vi "Lookup Command Info.vi"(8 "error in (no error)":errorcluster, 10 "Channel Lookup Info in":T4 {"Refs" format="%.0x"}, 11 "Item Ref in":T1 format="%.0x") -> (0 "error out":errorcluster, 1 "Command Parameters":T2, 2 "Channel Lookup Info out":T4 {"Refs" format="%.0x"}, 3 "Section Ref out":T1 format="%.0x")   [LabVIEW 2015, in "Instrument Addon System Explorer.lvlib"]
uses:
  Instrument Addon System Explorer.lvlib
  Types/Channel Lookup Cluster.ctl
  <vilib>/NI Veristand/Custom Device API/Custom Device Item Ref.ctl
  Shared/Types/Command Parameters.ctl
  Shared/Types/Linked Channel Cluster.ctl
  Shared/Types/FG Control.ctl
  Shared/MetaData Parameters FG.vi
  <vilib>/NI Veristand/Custom Device API/NI VeriStand - Get Item Property.vi
  <vilib>/NI Veristand/Custom Device API/Get Item Property (String).vi
  <vilib>/NI Veristand/Custom Device API/NI VeriStand - Set Item Property.vi
  <vilib>/NI Veristand/Custom Device API/Set Item Property (U32).vi
  <vilib>/NI Veristand/Custom Device API/Set Item Property (String).vi
  <vilib>/NI Veristand/Custom Device API/Set Item Property (String Array).vi
  <vilib>/NI Veristand/Custom Device API/Get Item Property (U32).vi
  <vilib>/NI Veristand/Custom Device API/Get Item Property (String Array).vi
  Shared/Constants.vi
  <vilib>/NI Veristand/Custom Device API/Set Item Property (Boolean).vi
  <vilib>/NI Veristand/Custom Device API/Get Item Property (Boolean).vi
  <vilib>/NI Veristand/Custom Device Tools/Custom Device Utility Library/NI VeriStand - Search for Item by GUID.vi
  <vilib>/NI Veristand/Custom Device Tools/Custom Device Utility Library/Custom Device Utility Library.lvlib
  Shared/Instrument Addon Shared.lvlib
  <vilib>/NI Veristand/Custom Device API/Custom Device API.lvlib
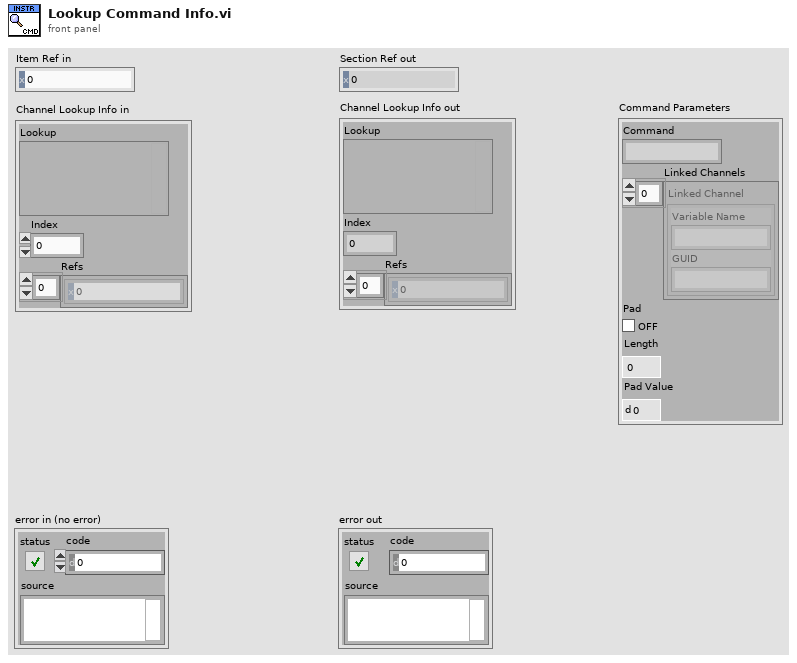
[diagram p1: front panel]
types:
  T1 = typedef "Custom Device API.lvlib/Custom Device Item Ref.ctl" = u64
  T2 = typedef "Instrument Addon Shared.lvlib/Command Parameters.ctl" = cluster{"Command":string, "Linked Channels":T3[], "Pad":bool, "Length":u32, "Pad Value":u8}
  T3 = typedef "Instrument Addon Shared.lvlib/Linked Channel Cluster.ctl" = cluster{"Variable Name":string, "GUID":string}
  T4 = typedef "Instrument Addon System Explorer.lvlib/Channel Lookup Cluster.ctl" = cluster{"Lookup":variant, "Index":i32, "Refs":T1[]}
  T5 = typedef "Instrument Addon Shared.lvlib/FG Control.ctl" = enum16{"Get", "Set"}
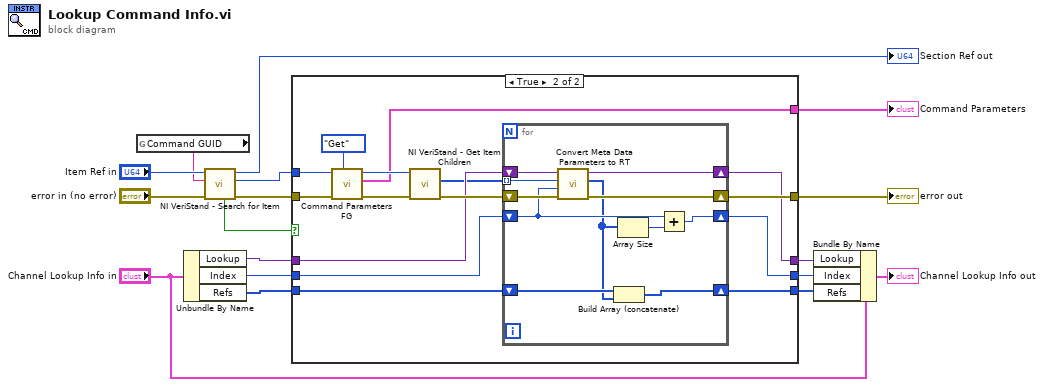
[diagram p0: block diagram]
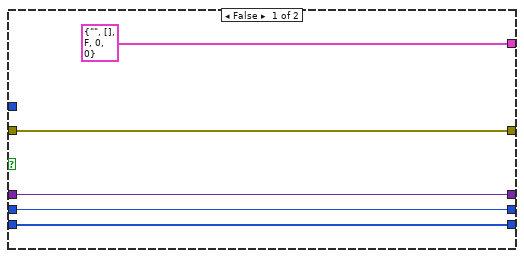
[diagram p2: hidden frame]
diagram:
  n1 = global read "Constants.vi" "Command GUID"() -> (w1:string)
  n2 = Unbundle By Name("Channel Lookup Info in") -> ("Lookup"=w10:variant, "Index"=w11:i32, "Refs"=w12:T1[])
  n3 = call-poly <vilib>:"NI VeriStand - Search for Item.vi"("error in"="error in (no error)", "Item GUID"=w1, "Section Ref in"="Item Ref in") -> ("error out"=w2:errorcluster, "Item Ref"=w4:T1, "Section Ref out"=→"Section Ref out":T1, "Found"=w7:bool)  [unwired: 5 in]
  n4 = case shown="True" w7 {
    tunnel: w2 -> [w22 w37]
    tunnel: [w22 w34] -> w3
    tunnel: w10 -> [w21 w31]
    tunnel: [w19 w23] -> w16
    tunnel: w12 -> [w19 w24]
    tunnel: w11 -> [w20 w29]
    tunnel: [w20 w28] -> w15
    tunnel: [w21 w27] -> w14
    tunnel: w4 -> [_ w26]
    tunnel: [T2 {"Command"="", "Linked Channels"=[], "Pad"=FALSE, "Length"=0, "Pad Value"=0} ("Command Parameters") w25] -> w6
    frame False {
    }
    frame True {
      n5 = call "Command Parameters FG.vi"("Action"=FG_Control."Get", "error in (no error)"=w37, "Item Ref in"=w26) -> ("error out"=w35:errorcluster, "Command Parameters"=w25:T2, "Item Ref out"=w32:T1)  [unwired: 6 in]
      n6 = call <vilib>:"NI VeriStand - Get Item Children.vi"("error in (no error)"=w35, "Item Ref in"=w32) -> ("error out"=w33:errorcluster, "Child Refs"=w30:T1[])  [unwired: 6 in, 2 out]
      n7 = for {
        shift-right: [w43] -> w34
        shift-left: w33 -> [w47]
        tunnel: w30 -> [w46] mode=indexing
        shift-right: [w48] -> w28
        shift-left: w29 -> [w41]
        shift-right: [w44] -> w27
        shift-left: w31 -> [w45]
        shift-right: [w39] -> w23
        shift-left: w24 -> [w40]
        n8 = call "Convert Meta Data Parameters to RT.vi"("error in (no error)"=w47, "Data Index"=w41, "Item Ref in"=w46, "Lookup Table"=w45) -> ("error out"=w43:errorcluster, "Chan Refs"=w38:T1[], "Lookup Table out"=w44:variant)  [unwired: 5 in]
        n9 = Build Array (concatenate)(w40, w38) -> (w39:T1[])
        n10 = Array Size(array=w38) -> (size(s)=w42:i32)
        n11 = Add(x=w41, y=w42) -> (x+y=w48:i32)
      }
    }
  }
  "Command Parameters" <- w6
  "error out" <- w3
  n12 = Bundle By Name(cluster="Channel Lookup Info in", "Lookup"=w14, "Index"=w15, "Refs"=w16) -> (→"Channel Lookup Info out":T4)
